vi "FPGAinit.vi"(4 "Testpulse Cluster":T2={"Master Pulser On/Off"=FALSE, "Testpulse Turnaround Time (samples)"=14, "Pulse Separation (samples)"=0, "Pulse duration (samples)"=0}, 5 "DAQ Info Cluster":T1={"Data Chunks per File"=1000, "Samples per Waveform"=95, "Pretrigger Samples"=15, "circular buffer length (samples)"=1000, "Waveforms per Data Chunk"=5000} {"Waveforms per Data Chunk" format="%.2p"}, 6 "Channel Cluster":T3={"det_type"=[], "voltage"=[], "Serial numbers"=[], "Sources"=[], "Trigger level"=[4000, 4000, 4000, 4000, 4000, 4000, 4000, 4000], "Channel On/Off"=[], "Number of Channels"=8}, 7 "General Cluster":cluster{"Location":i16} {"Location" items=["Purdue", "NIKHEF", "Zurich", "???"]}, 8 "error in":errorcluster, 11 "FPGA VI Reference In":refnum<k20>) -> (0 "error out":errorcluster, 3 "FPGA VI Reference Out":refnum<k20>)   [LabVIEW 2012]
uses:
  <vilib>/Utility/error.llb/Error Cluster From Error Code.vi
  <vilib>/LabVIEW Targets/FPGA/FlexRIO/CustomFPGAMethods/79XXR_Method_IOModuleStatusImpl.vi
  <vilib>/FPGAPlugInAG/Dynamic/niLvFpga_Run_Dynamic.vi
  <vilib>/rvi/errors/niLvFpgaAdjustHostInterfaceError.vi
  <vilib>/rvi/interface/nirviMethod/nirviMethod.xnode
  <vilib>/rvi/interface/nirviReadWriteControl/nirviReadWriteControl.xnode
  <vilib>/FPGAPlugInAG/Dynamic/niLvFpga_ConfigureFifo_Dynamic.vi
  <vilib>/rvi/errors/niLvFpgaMergeErrorWithErrorCode.vi
  <vilib>/FPGAPlugInAG/Dynamic/niLvFpga_StartFifo_Dynamic.vi
  NiFpgaLv.dll
  <vilib>/rvi/interface/Simulation/niFpgaSimulationCallBeginRW.vi
panel:
  # "Waveform/Data Chunk information"
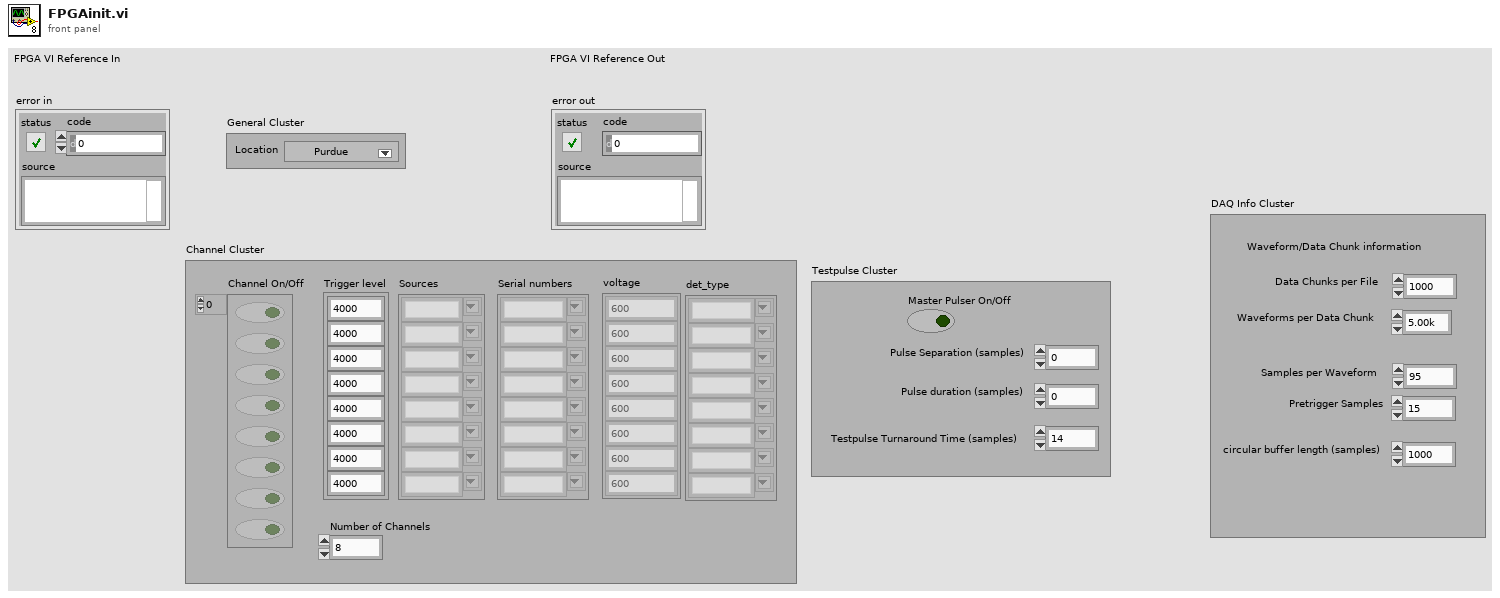
[diagram p1: front panel]
types:
  T1 = cluster{"Data Chunks per File":u32, "Samples per Waveform":u32, "Pretrigger Samples":u32, "circular buffer length (samples)":u32, "Waveforms per Data Chunk":u32}
  T2 = cluster{"Master Pulser On/Off":bool, "Testpulse Turnaround Time (samples)":u32, "Pulse Separation (samples)":u32, "Pulse duration (samples)":u32}
  T3 = cluster{"det_type":string[], "voltage":string[], "Serial numbers":string[], "Sources":string[], "Trigger level":i16[], "Channel On/Off":bool[], "Number of Channels":u8}
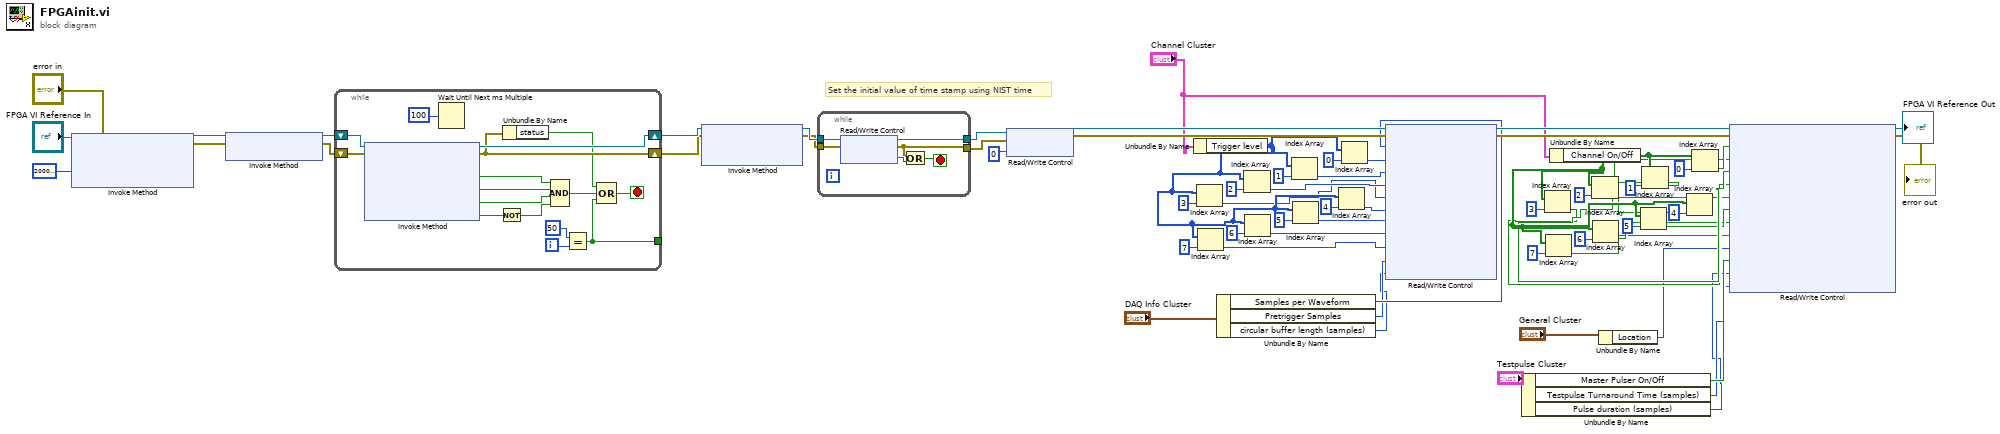
[diagram p0: block diagram]
diagram:
  # "Set the initial value of time stamp using NIST time"
  n1 = xnode "Invoke Method"("FPGA VI Reference In"="FPGA VI Reference In", "error in"="error in", "Requested Depth"=u32 20000000) -> ("FPGA VI Reference Out"=w64:refnum<k20>, "error out"=w65:errorcluster)  [unwired: 1 out]
  n2 = xnode "Invoke Method"("FPGA VI Reference In"=w64, "error in"=w65) -> ("FPGA VI Reference Out"=w43:refnum<k20>, "error out"=w42:errorcluster)
  n3 = while {
    shift-right: [w72] -> w59
    shift-left: w42 -> [w80]
    shift-right: [w79] -> w60
    shift-left: w43 -> [w81]
    tunnel: [w68] -> _
    i -> [w74]
    stop <- w69 stop-if-true
    n4 = xnode "Invoke Method"("FPGA VI Reference In"=w81, "error in"=w80) -> ("FPGA VI Reference Out"=w79:refnum<k20>, "error out"=w72:errorcluster, "IO Module Present?"=w78:bool, "Power Enabled?"=w77:bool, "IO Enabled?"=w76:bool, "IO Module Mismatch?"=w67:bool)
    n5 = Wait Until Next ms Multiple(millisecond multiple=u32 100) -> ()  [unwired: 1 out]
    n6 = Not(x=w67) -> (.not. x?=w66:bool)
    n7 = Unbundle By Name(w72) -> ("status"=w71:bool)
    n8 = Compound Arithmetic op=AND(w78, w77, w76, w66) -> (w70:bool)
    n9 = Equal?(x=50, y=w74) -> (x = y?=w68:bool)
    n10 = Compound Arithmetic op=OR(w71, w70, w68) -> (w69:bool)
  }
  n11 = xnode "Invoke Method"("FPGA VI Reference In"=w60, "error in"=w59) -> ("FPGA VI Reference Out"=w62:refnum<k20>, "error out"=w61:errorcluster)  [unwired: 1 in]
  n12 = while {
    tunnel: [w82] -> w57
    tunnel: [w87] -> w58
    tunnel: w62 -> [w86]
    tunnel: w61 -> [w85]
    stop <- w83 stop-if-true
    n13 = xnode "Read/Write Control"("FPGA VI Reference In"=w86, "error in"=w85) -> ("FPGA VI Reference Out"=w87:refnum<k20>, "error out"=w82:errorcluster, "Init Done"=w84:bool)
    n14 = Or(x=w82, y=w84) -> (x .or. y?=w83:bool)
  }
  n15 = xnode "Read/Write Control"("FPGA VI Reference In"=w58, "error in"=w57, "initial value"=u64 0) -> ("FPGA VI Reference Out"=w45:refnum<k20>, "error out"=w46:errorcluster)
  n16 = Unbundle By Name("Channel Cluster") -> ("Trigger level"=w41:i16[])
  n17 = Index Array(array=w41, index=3) -> (element=w37:i16)
  n18 = Index Array(array=w41, index=7) -> (element=w33:i16)
  n19 = Unbundle By Name("DAQ Info Cluster") -> ("Samples per Waveform"=w3:u32, "Pretrigger Samples"=w2:u32, "circular buffer length (samples)"=w1:u32)
  n20 = Index Array(array=w41, index=2) -> (element=w38:i16)
  n21 = Index Array(array=w41, index=6) -> (element=w34:i16)
  n22 = Index Array(array=w41, index=1) -> (element=w39:i16)
  n23 = Index Array(array=w41, index=5) -> (element=w35:i16)
  n24 = Index Array(array=w41, index=4) -> (element=w36:i16)
  n25 = Index Array(array=w41, index=0) -> (element=w40:i16)
  n26 = xnode "Read/Write Control"("FPGA VI Reference In"=w45, "error in"=w46, "Record Size only data"=w3, "Trigger 0"=w40, "Trigger 1"=w39, "Trigger 2"=w38, "Trigger 3"=w37, "Trigger 4"=w36, "Trigger 5"=w35, "Trigger 6"=w34, "Trigger 7"=w33, "# of pretrigger"=w2, "circular buffer length"=w1) -> ("FPGA VI Reference Out"=w54:refnum<k20>, "error out"=w55:errorcluster)
  n27 = Unbundle By Name("Testpulse Cluster") -> ("Master Pulser On/Off"=w8:bool, "Testpulse Turnaround Time (samples)"=w6:u32, "Pulse duration (samples)"=w5:u32)
  n28 = Unbundle By Name("Channel Cluster") -> ("Channel On/Off"=w25:bool[])
  n29 = Index Array(array=w25, index=3) -> (element=w21:bool)
  n30 = Index Array(array=w25, index=7) -> (element=w17:bool)
  n31 = Index Array(array=w25, index=2) -> (element=w22:bool)
  n32 = Index Array(array=w25, index=6) -> (element=w18:bool)
  n33 = Unbundle By Name("General Cluster") -> ("Location"=w7:i16)
  n34 = Index Array(array=w25, index=5) -> (element=w19:bool)
  n35 = Index Array(array=w25, index=1) -> (element=w23:bool)
  n36 = Index Array(array=w25, index=4) -> (element=w20:bool)
  n37 = Index Array(array=w25, index=0) -> (element=w24:bool)
  n38 = xnode "Read/Write Control"("FPGA VI Reference In"=w54, "error in"=w55, "channel 0 on/off"=w24, "channel 1 on/off"=w23, "channel 2 on/off"=w22, "channel 3 on/off"=w21, "channel 4 on/off"=w20, "channel 5 on/off"=w19, "channel 6 on/off"=w18, "channel 7 on/off"=w17, "location"=w7, "Testpulser On/Off"=w8, "Testpulse duration (20 ns ticks)"=w5, "Testpulse Time Delay (20 ns ticks)"=w6) -> ("FPGA VI Reference Out"=→"FPGA VI Reference Out":refnum<k20>, "error out"=→"error out":errorcluster)
